vi "Copy sheet 1 to sheet 2.vi"(0 "Excel._Workbook":refnum<k7>, 5 "Work Sheet":refnum<k7>, 7 "WorkSheets":refnum<k7>, 9 "Write/Read Cell":T1={"Cell Range"="", "Data 2D"=[], "Select Sheet"="", "1 Data"="", "Data 1D"=[], "Font col"=0, "Bold"=TRUE, "Font Size"=18, "Inside lines"=FALSE}, 11 "error in":errorcluster) -> (4 "Excel._Workbook":refnum<k7>, 6 "Work Sheet":refnum<k7>, 15 "error out":errorcluster)   [LabVIEW 2017]
uses:
  controls/read.write.ctl
panel:
  out "Worksheets":refnum<k7>
  in  "Excel._Worksheet":refnum<k7>
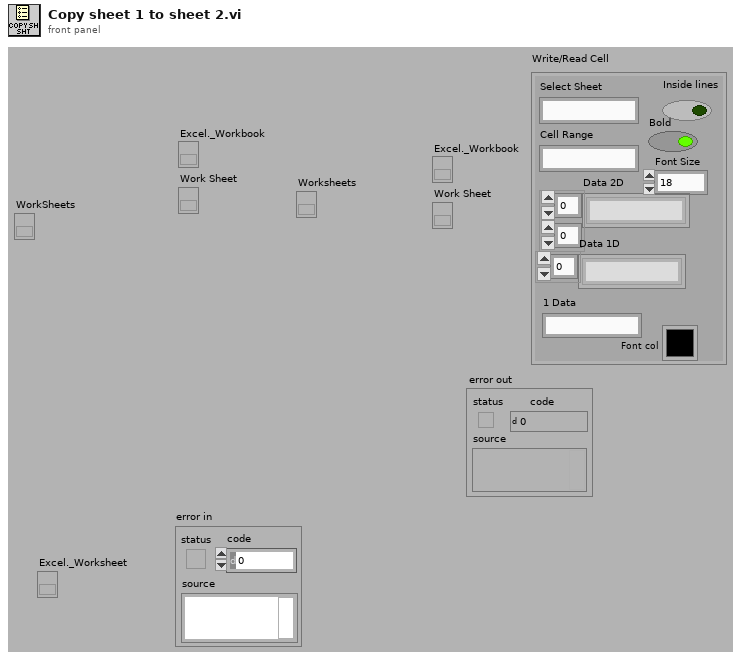
[diagram p1: front panel]
types:
  T1 = typedef "read.write.ctl" = cluster{"Cell Range":string, "Data 2D":string[][], "Select Sheet":string, "1 Data":string, "Data 1D":string[], "Font col":u32, "Bold":bool, "Font Size":i32, "Inside lines":bool}
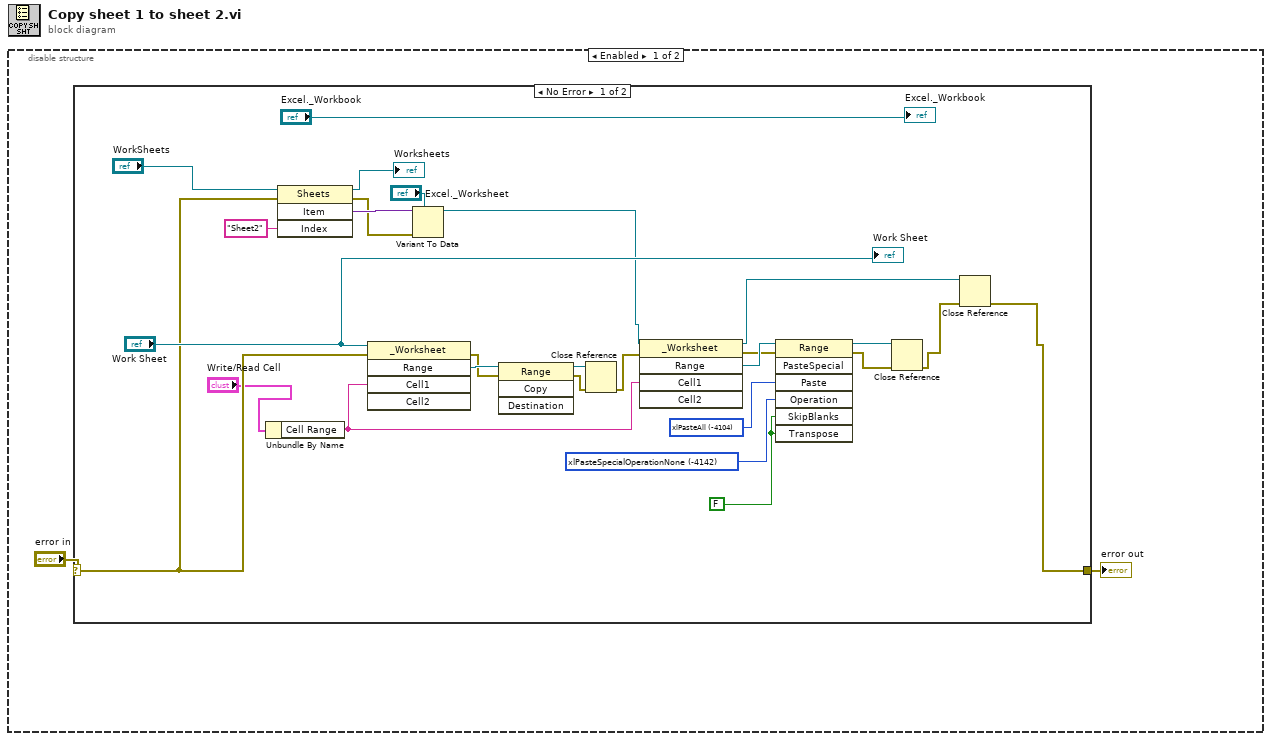
[diagram p0: block diagram]
diagram:
  n1 = disable-structure shown="Enabled" {
    frame Enabled {
      n2 = case shown="No Error" "error in" {
        selector: "error in" -> [w5 w30]
        tunnel: [w13 w30] -> w1
        frame No Error {
          w17 = FALSE
          w23 = -4142 items=["xlPasteSpecialOperationAdd"=2, "xlPasteSpecialOperationDivide"=5, "xlPasteSpecialOperationMultiply"=4, "xlPasteSpecialOperationNone"=-4142, "xlPasteSpecialOperationSubtract"=3] ("Operation")
          w24 = -4104 items=["xlPasteAll"=-4104, "xlPasteAllExceptBorders"=7, "xlPasteFormats"=-4122, "xlPasteFormulas"=-4123, "xlPasteComments"=-4144, "xlPasteValues"=-4163, "xlPasteColumnWidths"=8, "xlPasteValidation"=6, "xlPasteFormulasAndNumberFormats"=11, "xlPasteValuesAndNumberFormats"=12] ("Paste")
          n3 = Unbundle By Name("Write/Read Cell") -> ("Cell Range"=w12:string)
          n4 = invoke class="Sheets" method="Item"(reference="WorkSheets", error in=w5, "Index"="Sheet2" ("Sheet Name")) -> (reference out=→"Worksheets":refnum<k7>, error out=w10:errorcluster, "Item"=w11:variant)  [unwired: 1 in, 1 out]
          n5 = invoke class="_Worksheet" method="Range"(reference="Work Sheet", error in=w5, "Cell1"=w12) -> (error out=w27:errorcluster, "Range"=w28:refnum<k7>)  [unwired: 2 in, 3 out]
          n6 = Variant To Data(error in=w10, type="Excel._Worksheet", Variant=w11) -> (data=w4:refnum<k7>)  [unwired: 1 out]
          n7 = invoke class="Range" method="Copy"(reference=w28, error in=w27) -> (reference out=w26:refnum<k7>, error out=w20:errorcluster)  [unwired: 2 in, 2 out]
          n8 = Close Reference(reference=w26, error in (no error)=w20) -> (error out=w19:errorcluster)
          n9 = invoke class="_Worksheet" method="Range"(reference=w4, error in=w19, "Cell1"=w12) -> (reference out=w15:refnum<k7>, error out=w21:errorcluster, "Range"=w25:refnum<k7>)  [unwired: 2 in, 2 out]
          n10 = invoke class="Range" method="PasteSpecial"(reference=w25, error in=w21, "Paste"=w24, "Operation"=w23, "SkipBlanks"=w17, "Transpose"=w17) -> (reference out=w22:refnum<k7>, error out=w18:errorcluster)  [unwired: 1 in, 5 out]
          n11 = Close Reference(reference=w22, error in (no error)=w18) -> (error out=w14:errorcluster)
          n12 = Close Reference(reference=w15, error in (no error)=w14) -> (error out=w13:errorcluster)
          "Work Sheet" <- "Work Sheet"
          "Excel._Workbook" <- "Excel._Workbook"
        }
        frame Error {
        }
      }
      "error out" <- w1
    }
    frame Disabled {
    }
  }
